vi "VisionAssistanceFinal.vi"() -> ()   [LabVIEW 2019]
uses:
  <vilib>/vision/Image Controls.llb/IMAQ Image.ctl
panel:
  out "error out":errorcluster
  out "sorted circles by center x then y":T1(array[cluster])
  in  "Circle Descriptor (Shape Detection 1)":cluster{"Min Radius":dbl, "Max Radius":dbl}={"Min Radius"=30.0, "Max Radius"=300.0}
  in  "read image\nalgorithm":bool=TRUE
  out "i":i32
  out "Image Out":T2(plugin-control)
  in  "stop Control?":bool
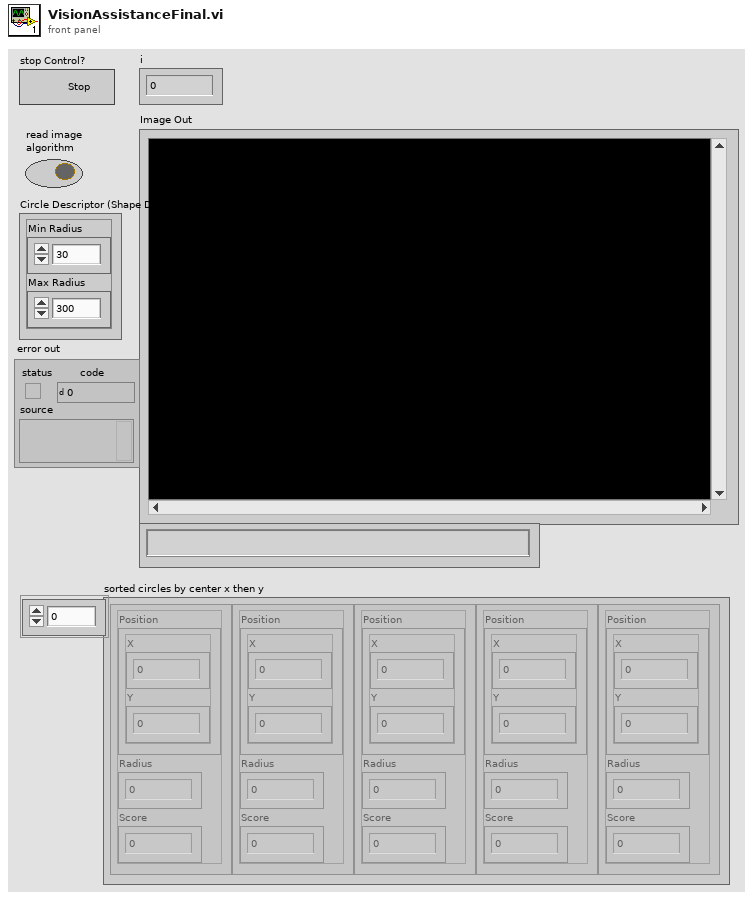
[diagram p1: front panel]
types:
  T1 = cluster{"Position":cluster{"X":u16, "Y":u16}, "Radius":u16, "Score":u16}[]
  T2 = typedef "IMAQ Image.ctl" = refnum<image>
  T3 = typedef "Image Type" = u32
  T4 = cluster{"Position":cluster{"X":sgl, "Y":sgl}, "Radius":dbl, "Score":dbl}[]
  T5 = cluster{"Position":cluster{"X":u16, "Y":u16}, "Radius":u16, "Score":u16}
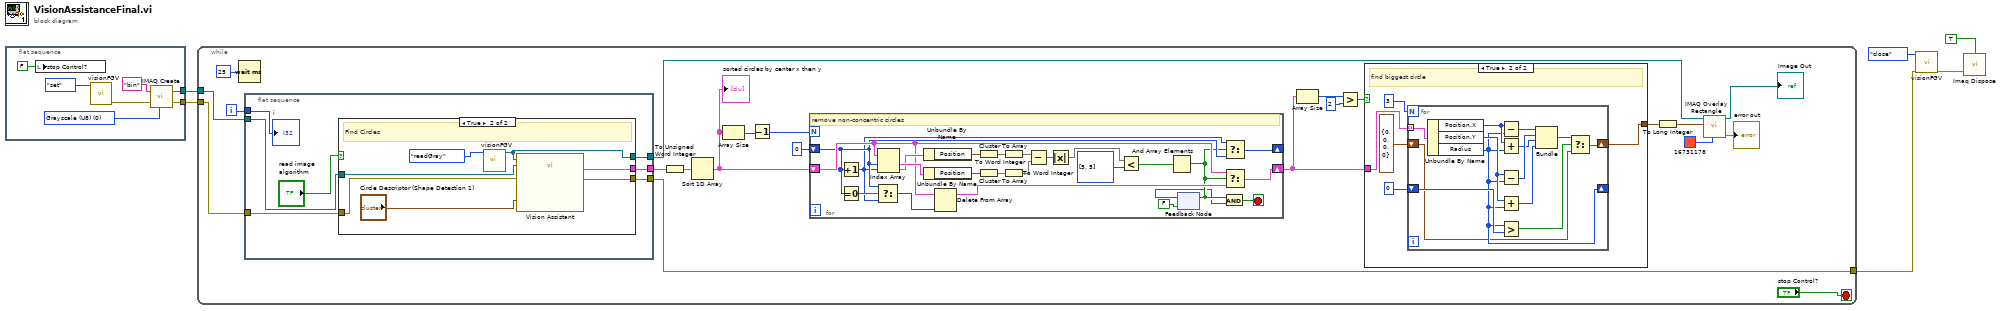
[diagram p0: block diagram]
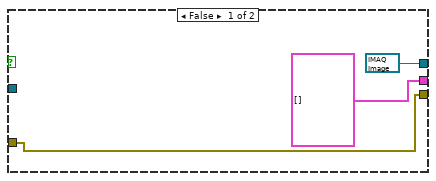
[diagram p2: hidden frame]
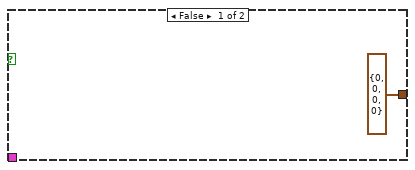
[diagram p3: hidden frame]
diagram:
  n1 = flat-sequence {
    tunnel: [w12] -> w6
    tunnel: [w9] -> w3
    frame #0 {
      w11 = T3 0 items=["Grayscale (U8)", "Grayscale (I16)", "Grayscale (SGL)", "Complex (CSG)", "RGB (U32)", "HSL (U32)", "RGB (U64)", "Grayscale (U16)"] ("Image Type")
      n2 = local write "stop Control?"(FALSE ("stop Control?")) -> ()
      n3 = call "visionFGV.vi"("Function"=enum16{"set", "readColor", "close", "readGray"}."set") -> ("error out"=w7:errorcluster)  [unwired: 9 in, 1 out]
      n4 = call "IMAQ Create"("Image Name"="bin", "Image Type"=w11, "error in (no error)"=w7) -> ("New Image"=w12:T2, "error out"=w9:errorcluster)  [unwired: 2 in]
    }
  }
  n5 = while {
    tunnel: [w25] -> w2
    tunnel: w6 -> [w34]
    tunnel: w3 -> [w19]
    i -> [w30]
    stop <- "stop Control?" stop-if-true
    n6 = Wait (ms)(milliseconds to wait=u32 25) -> ()  [unwired: 1 out]
    n7 = flat-sequence {
      tunnel: [w40] -> w25
      tunnel: [w38] -> w22
      tunnel: [w36] -> w18
      tunnel: w34 -> [w42]
      tunnel: w30 -> [w41]
      tunnel: w19 -> [w37]
      frame #0 {
        n8 = case shown="True" "read image\nalgorithm" {
          tunnel: [w44 w50] -> w40
          tunnel: w42 -> [_ w52]
          tunnel: [T4 [] ("Circles (Shape Detection 1)") w51] -> w38
          tunnel: w37 -> [w44 w48]
          tunnel: [T2 refnum ("Image Out fgv") w46] -> w36
          frame False {
          }
          frame True {
            # "Find Circles"
            n9 = call "visionFGV.vi"("Function"=enum16{"set", "readColor", "close", "readGray"}."readGray") -> ("Image Out fgv"=w46:T2)  [unwired: 9 in, 1 out]
            n10 = call "Vision Assistant"("Image In"=w46, "Image Dst"=w52, "Circle Descriptor (Shape Detection 1)"="Circle Descriptor (Shape Detection 1)", "error in"=w48) -> ("Circles (Shape Detection 1)"=w51:T4, "error out"=w50:errorcluster)  [unwired: 21 in, 1 out]
          }
        }
        "i" <- w41
      }
    }
    n11 = To Unsigned Word Integer(number=w22) -> (unsigned 16bit integer=w29:T1)
    n12 = Sort 1D Array(array=w29) -> (sorted array=w26:T1)
    "sorted circles by center x then y" <- w26
    n13 = Array Size(array=w26) -> (size(s)=w28:i32)
    n14 = Decrement(x=w28) -> (x-1=w27:i32)
    n15 = for {
      N: w27 -> [_]
      shift-right: [w72] -> w23
      shift-left: w26 -> [w71]
      shift-right: [w70] -> _
      shift-left: 0 ("index") -> [w67]
      stop <- w61 stop-if-true
      # "remove non-concentric circles"
      n16 = Increment(x=w67) -> (x+1=w65:i32)
      n17 = Equal To 0?(x=w67) -> (x = 0?=w68:bool)
      n18 = Select(t=w67, s=w68, f=w65) -> (s? t:f=w66:i32)
      n19 = Index Array(array=w71, index #1=w67, index #2=w65) -> (element #1=w76:T5, element #2=w74:T5)
      n20 = Unbundle By Name(w74) -> ("Position"=w73:cluster{"X":u16, "Y":u16})
      n21 = Unbundle By Name(w76) -> ("Position"=w75:cluster{"X":u16, "Y":u16})
      n22 = Delete From Array(array=w71, index=w66) -> (array with subset deleted=w69:T1)  [unwired: 1 in, 1 out]
      n23 = Cluster To Array(cluster=w73) -> (array=w60:u16[])
      n24 = Cluster To Array(cluster=w75) -> (array=w59:u16[])
      n25 = To Word Integer(number=w60) -> (16bit integer=w57:i16[])
      n26 = To Word Integer(number=w59) -> (16bit integer=w58:i16[])
      n27 = Subtract(x=w57, y=w58) -> (x-y=w56:i16[])
      n28 = Absolute Value(x=w56) -> (abs(x)=w55:i16[])
      n29 = Less?(x=w55, y=i16[] [5, 5]) -> (x < y?=w53:bool[])
      n30 = And Array Elements(Boolean array=w53) -> (logical AND=w64:bool)
      n31 = feedback-in #1(w64) -> ()
      n32 = feedback #1(FALSE) -> (w63:bool)
      n33 = And(x=w64, y=w63) -> (x .and. y?=w61:bool)
      n34 = Select(t=w65, s=w64, f=w67) -> (s? t:f=w70:i32)
      n35 = Select(t=w71, s=w64, f=w69) -> (s? t:f=w72:T1)
    }
    n36 = Array Size(array=w23) -> (size(s)=w33:i32)
    n37 = Greater?(x=w33, y=2) -> (0:w15:bool)
    n38 = case shown="True" w15 {
      tunnel: w23 -> [_ w80]
      tunnel: [cluster{u16, u16, u16, u16} {0, 0, 0, 0} ("f") w82] -> w20
      frame False {
      }
      frame True {
        # "find biggest circle"
        n39 = for {
          N: 3 ("index") -> [_]
          tunnel: w80 -> [w88] mode=indexing
          shift-right: [w83] -> w82
          shift-left: cluster{u16, u16, u16, u16} {0, 0, 0, 0} -> [w84]
          shift-right: [w85] -> _
          shift-left: u16 0 ("Radius") -> [w86]
          n40 = Unbundle By Name(w88) -> ("Position.X"=w93:u16, "Position.Y"=w91:u16, "Radius"=w85:u16)
          n41 = Subtract(x=w93, y=w85) -> (x-y=w95:u16)
          n42 = Add(x=w93, y=w85) -> (x+y=w92:u16)
          n43 = Subtract(x=w91, y=w85) -> (x-y=w94:u16)
          n44 = Add(x=w91, y=w85) -> (x+y=w90:u16)
          n45 = Greater?(x=w85, y=w86) -> (0:w89:bool)
          n46 = Bundle(w95, w94, w92, w90) -> (w87:cluster{u16, u16, u16, u16})  [unwired: 1 in]
          n47 = Select(t=w87, s=w89, f=w84) -> (s? t:f=w83:cluster{u16, u16, u16, u16})
        }
      }
    }
    n48 = To Long Integer(number=w20) -> (32bit integer=w21:cluster{i32, i32, i32, i32})
    n49 = call "IMAQ Overlay Rectangle"("Color"=u32 16731178, "Rectangle"=w21, "Image"=w18) -> ("error out"=→"error out":errorcluster, "Image Out"=→"Image Out":T2)  [unwired: 7 in]
  }
  n50 = call "visionFGV.vi"("Error In"=w2, "Function"=enum16{"set", "readColor", "close", "readGray"}."close") -> ("error out"=w1:errorcluster)  [unwired: 8 in, 1 out]
  n51 = call "Imaq Dispose"("All Images? (No)"=TRUE, "error in (no error)"=w1) -> ()  [unwired: 4 in, 1 out]
